vi "CRYExport to Excel with Close.vi"(4 "Format info":T1, 6 "ExcelPath":string, 8 "FilePath":string, 9 "Sheet Names":string[](array[string]), 10 "Data":string[][][](array[string]), 11 "New/Append":string) -> (0 "error out":errorcluster)   [LabVIEW 2013]
uses:
  <vilib>/addons/_office/_exclsub.llb/font.ctl
  <vilib>/Utility/NIReport.llb/NI_report.lvclass
  <vilib>/addons/_office/excel.llb/Excel Easy Table (str).vi
  <vilib>/Utility/NIReport.llb/Excel/NI_Excel.lvclass
  <vilib>/addons/_office/NI_ReportGenerationToolkit.lvlib
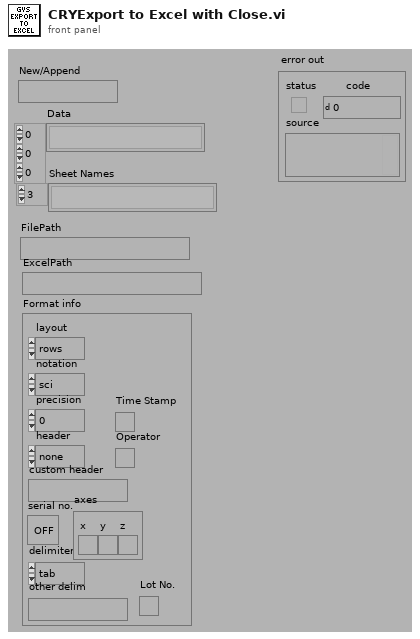
[diagram p1: front panel]
types:
  T1 = cluster{"layout":enum16{"rows", "columns"}, "notation":enum16{"sci", "float"}, "precision":i32, "header":enum16{"none", "standard", "custom"}, "custom header":string, "serial no.":bool, "delimiter":enum16{"tab", "comma", "space", "other"}, "other delim":string, "axes":cluster{"x":bool, "y":bool, "z":bool}, "Lot No.":bool, "Operator":bool, "Time Stamp":bool}
  T2 = typedef "NI_ReportGenerationToolkit.lvlib/font.ctl" = cluster{"font name":string, "font size":dbl, "bold":u16, "italic":u16, "underline":u16, "strike through":u16, "font color":u32}
  T3 = enum16{"OK", "Yes", "YesNo", "YesNoCancel", "ReplaceAppend"}
  T4 = enum16{"maximized", "minimized", "normal", "no change"}
  T5 = enum16{"Standard Report", "HTML", "Word", "Excel"}
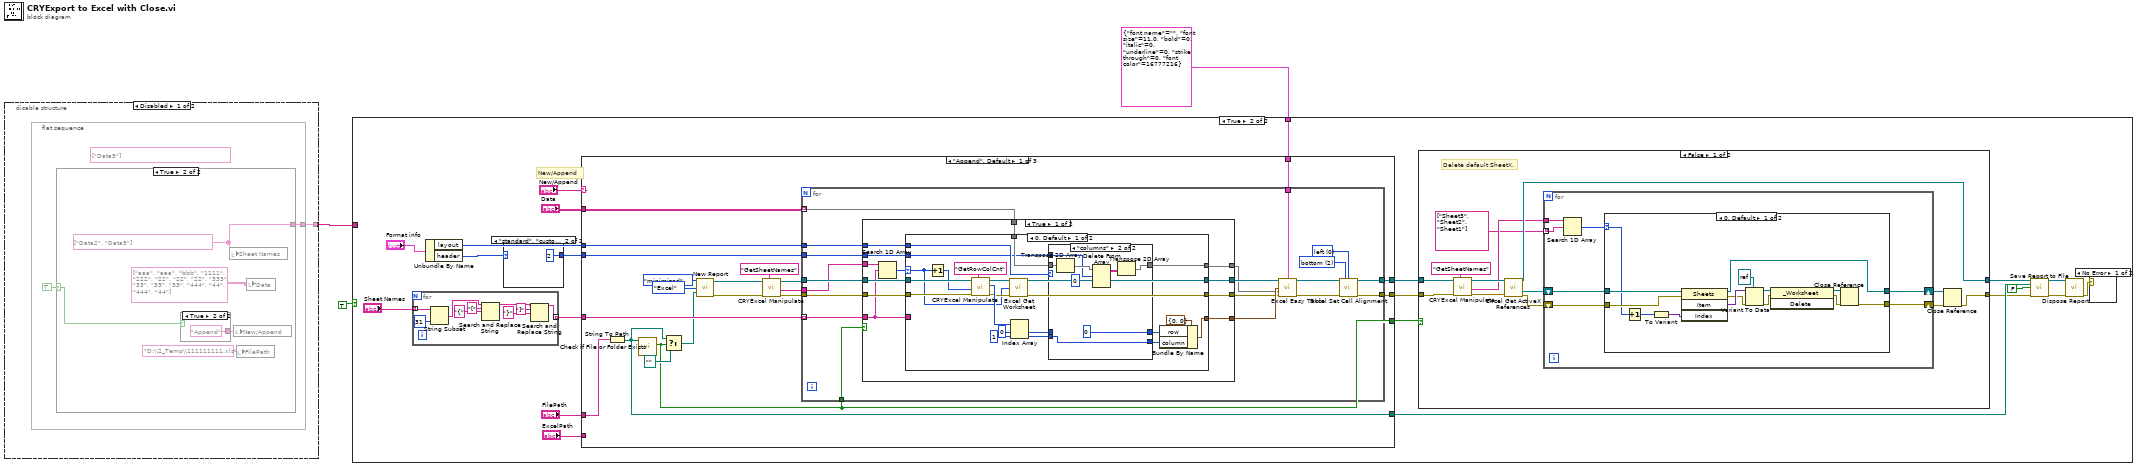
[diagram p0: block diagram]
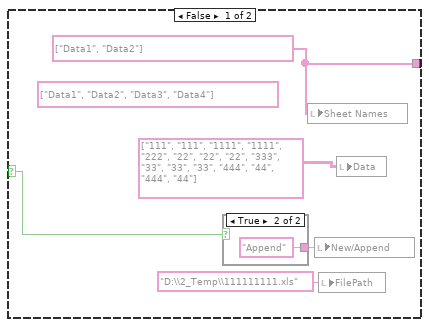
[diagram p2: hidden frame]
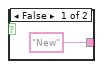
[diagram p3: hidden frame]
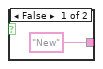
[diagram p4: hidden frame]
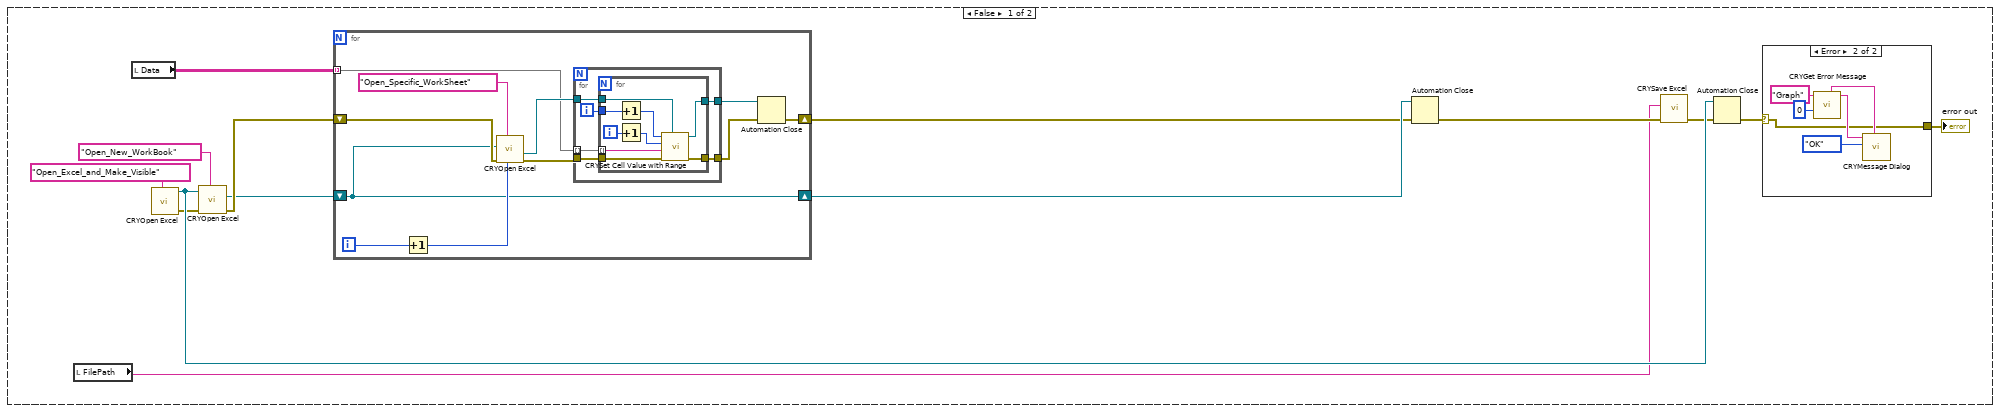
[diagram p6: hidden frame]
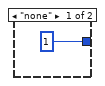
[diagram p8: hidden frame]
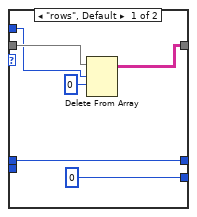
[diagram p12: hidden frame]
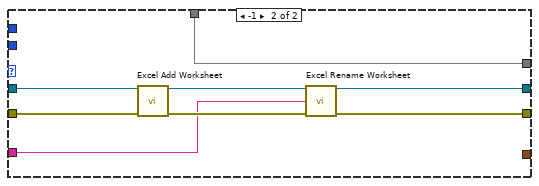
[diagram p13: hidden frame]
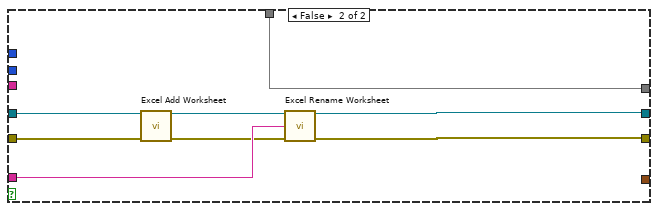
[diagram p14: hidden frame]
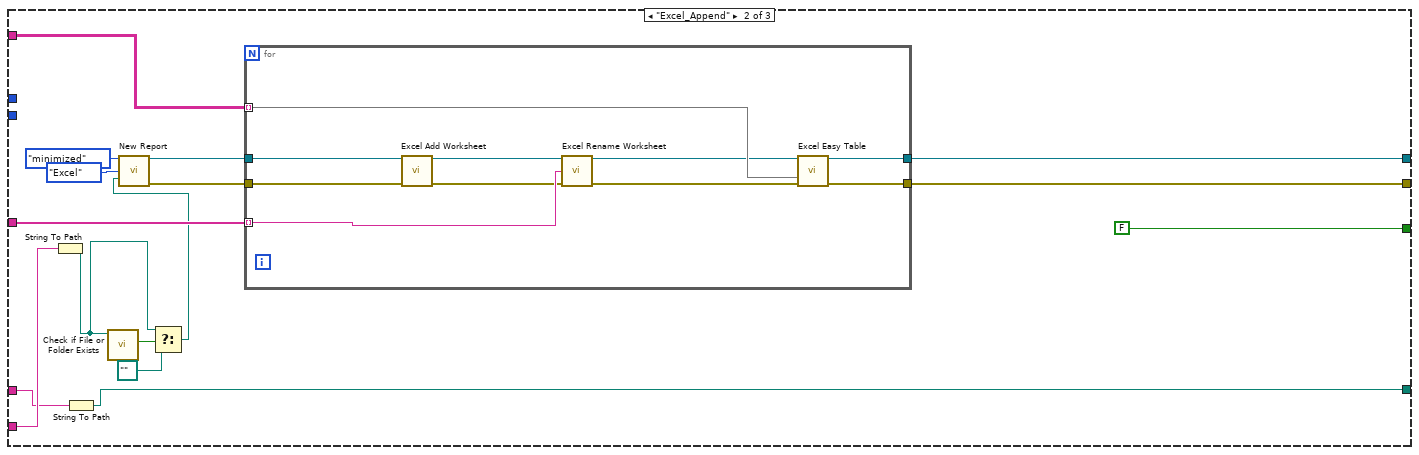
[diagram p15: hidden frame]
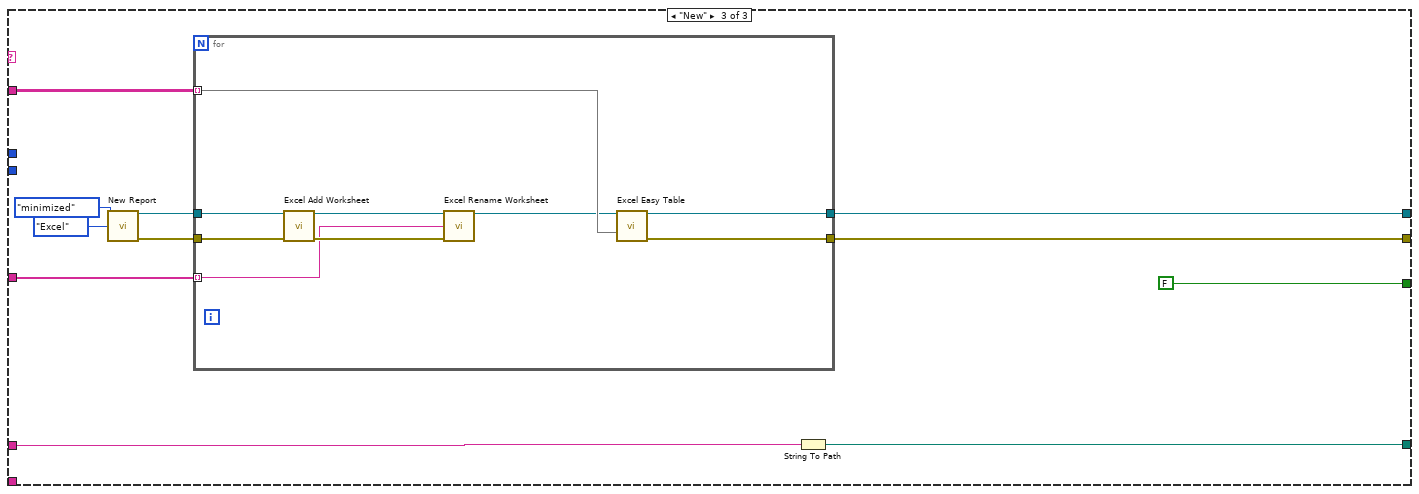
[diagram p16: hidden frame]
diagram:
  n1 = disable-structure shown="Disabled" {
    disable-tunnel: [w4 _] -> w2
    frame Disabled {
      n2 = flat-sequence {
        tunnel: [w6] -> w4
        frame #0 {
          (unwired) string[] ["Data5"] ("Data Names")
          n3 = case shown="True" TRUE {
            selector: TRUE -> [w8 w14]
            tunnel: [w7 w18] -> w6
            frame False {
              w7 = string[] ["Data1", "Data2"] ("Data Names")
              (unwired) string[] ["Data1", "Data2", "Data3", "Data4"] ("Data Names")
              n4 = case shown="True" w8 {
                tunnel: ["New" ("New/Append") "Append" ("New/Append")] -> w10
                frame False {
                }
                frame True {
                }
              }
              n5 = local write "Sheet Names"(w7) -> ()
              n6 = local write "New/Append"(w10) -> ()
              n7 = local write "FilePath"("D:\\2_Temp\\111111111.xls" ("FilePath")) -> ()
              n8 = local write "Data"(string[][][] [[["111", "111"], ["1111", "1111"]], [["222", "22"], ["22", "22"]], [["333", "33"], ["33", "33"]], [["444", "44"], ["444", "44"]]] ("appended array")) -> ()
            }
            frame True {
              w18 = string[] ["Data2", "Data5"] ("Data Names")
              n9 = case shown="True" w14 {
                tunnel: ["New" ("New/Append") "Append" ("New/Append")] -> w16
                frame False {
                }
                frame True {
                }
              }
              n10 = local write "Sheet Names"(w18) -> ()
              n11 = local write "New/Append"(w16) -> ()
              n12 = local write "FilePath"("D:\\2_Temp\\111111111.xls" ("FilePath")) -> ()
              n13 = local write "Data"(string[][][] [[["aaa", "aaa"], ["bbb", "1111"]], [["222", "22"], ["22", "22"]], [["333", "33"], ["33", "33"]], [["444", "44"], ["444", "44"]]] ("appended array")) -> ()
            }
          }
        }
      }
    }
    frame Enabled {
    }
  }
  n14 = case shown="True" TRUE {
    tunnel: w2 -> [_ _]
    tunnel: T2 {"font name"="", "font size"=11.0, "bold"=0, "italic"=0, "underline"=0, "strike through"=0, "font color"=16777216} ("font") -> [_ w72]
    frame False {
      n15 = local read "FilePath"() -> (w21:string)
      n16 = local read "Data"() -> (w22:string[][][])
      n17 = call "CRYOpen Excel.vi"("sActon"="Open_Excel_and_Make_Visible") -> ("error out"=w29:errorcluster, "Excel._Application out"=w32:refnum<k7>)  [unwired: 7 in, 2 out]
      n18 = call "CRYOpen Excel.vi"("sActon"="Open_New_WorkBook", "error in (no error)"=w29, "Excel._Application"=w32) -> ("error out"=w34:errorcluster, "Excel._Worksheets out"=w33:refnum<k7>)  [unwired: 5 in, 2 out]
      n19 = for {
        tunnel: w22 -> [w41] mode=indexing
        shift-right: [w35] -> w24
        shift-left: w34 -> [w45]
        shift-right: [w38] -> w25
        shift-left: w33 -> [w38]
        i -> [w40]
        n20 = Increment(x=w40) -> (x+1=w39:i32)
        n21 = call "CRYOpen Excel.vi"("Numeric"=w39, "sActon"="Open_Specific_WorkSheet", "error in (no error)"=w45, "Excel._Worksheets"=w38) -> ("error out"=w44:errorcluster, "Excel._Worksheet out"=w43:refnum<k7>)  [unwired: 4 in, 2 out]
        n22 = for {
          tunnel: w43 -> [w51]
          tunnel: w44 -> [w49]
          tunnel: [w48] -> w37
          tunnel: [w47] -> w36
          tunnel: w41 -> [w46] mode=indexing
          i -> [w50]
          n23 = for {
            tunnel: w51 -> [w59]
            tunnel: w49 -> [w58]
            tunnel: [w57] -> w47
            tunnel: w50 -> [w56]
            tunnel: [w55] -> w48
            tunnel: w46 -> [w52] mode=indexing
            i -> [w60]
            n24 = Increment(x=w56) -> (x+1=w54:i32)
            n25 = Increment(x=w60) -> (x+1=w53:i32)
            n26 = call "CRYSet Cell Value with Range.vi"("Excel._Worksheet"=w59, "error in (no error)"=w58, "Value"=w52, "Col"=w53, "Row"=w54) -> ("error out"=w57:errorcluster, "Excel._Worksheet"=w55:refnum<k7>)  [unwired: 2 out]
          }
        }
        n27 = Automation Close(3:w36, 5:w37) -> (0:w35:errorcluster)
      }
      n28 = Automation Close(3:w24, 5:w25) -> (0:w28:errorcluster)
      n29 = call "CRYSave Excel.vi"("error in (no error)"=w28, "FilePath"=w21) -> ("error out"=w27:errorcluster)  [unwired: 8 in]
      n30 = Automation Close(3:w27, 5:w32) -> (0:w26:errorcluster)
      n31 = case shown="Error" w26 {
        selector: w26 -> [w61 w62]
        tunnel: [w61 w62] -> w23
        frame No Error {
        }
        frame Error {
          n32 = call "CRYGet Error Message.vi"("Error No"=0, "Kind"="Graph") -> ("Message"=w64:string, "Window Title"=w63:string)  [unwired: 4 in, 4 out]
          n33 = call "CRYMessage Dialog.vi"("Window Title"=w63, "YesNoCancel"=T3."OK", "Message Content"=w64) -> ()  [unwired: 7 in, 2 out]
        }
      }
      "error out" <- w23
    }
    frame True {
      # "New/Append"
      n34 = for {
        tunnel: "Sheet Names" -> [w132] mode=indexing
        tunnel: [w129] -> w83 mode=indexing
        n35 = String Subset(string=w132, length (rest)=31 ("length (rest)")) -> (substring=w130:string)  [unwired: 1 in]
        n36 = Search and Replace String(input string=w130, search string="[", replace string="{" ("replace string (\"\")")) -> (result string=w133:string)  [unwired: 5 in, 3 out]
        n37 = Search and Replace String(input string=w133, search string="]", replace string="}" ("replace string (\"\")")) -> (result string=w129:string)  [unwired: 5 in, 3 out]
      }
      n38 = Unbundle By Name("Format info") -> ("layout"=w70:enum16{"rows", "columns"}, "header"=w69:enum16{"none", "standard", "custom"})
      n39 = case shown="\"standard\", \"custom\", Default" w69 {
        tunnel: [1 ("length") 2 ("length")] -> w68
        frame "none" {
        }
        frame "standard", "custom", Default {
        }
      }
      n40 = case shown="\"Append\", Default" "New/Append" {
        tunnel: "Data" -> [w156 w253 w274]
        tunnel: w83 -> [w155 w252 w273]
        tunnel: "FilePath" -> [w153 w247 w272]
        tunnel: "ExcelPath" -> [_ w248 _]
        tunnel: [w150 w243 w271] -> w79
        tunnel: [w149 w245 w270] -> w78
        tunnel: [w148 w244 w269] -> w77
        tunnel: [w151 FALSE ("file or folder exists?") FALSE] -> w74
        tunnel: w70 -> [w144 _ _]
        tunnel: w72 -> [w140 _ _]
        tunnel: w68 -> [w139 _ _]
        frame "Append", Default {
          n41 = String To Path(string=w153) -> (path=w150:path)
          n42 = call <vilib>:"Check if File or Folder Exists.vi"("path"=w150) -> ("file or folder exists?"=w151:bool)  [unwired: 8 in, 2 out]
          n43 = Select(t=w150, s=w151, f=path "") -> (s? t:f=w152:path)
          n44 = call <vilib>:"New Report.vi"("window state (normal)"=T4."minimized", "report type"=T5."Excel", "template (empty)"=w152) -> ("report out"=w143:refnum<class "NI_report.lvclass">, "error out"=w141:errorcluster)  [unwired: 3 in, 8 out]
          n45 = call "CRYExcel Manipulate.vi"("sAction"="GetSheetNames", "error in (no error)"=w141, "report in"=w143) -> ("error out"=w146:errorcluster, "sData out"=w145:string[], "report out"=w142:refnum<class "NI_report.lvclass">)  [unwired: 5 in, 1 out]
          n46 = for {
            tunnel: w142 -> [w176]
            tunnel: w146 -> [w175]
            tunnel: [w162] -> w149
            tunnel: [w160] -> w148
            tunnel: w156 -> [w167] mode=indexing
            tunnel: w155 -> [w174] mode=indexing
            tunnel: w151 -> [w173]
            tunnel: w145 -> [w172]
            tunnel: w144 -> [w168]
            tunnel: w140 -> [w165]
            tunnel: w139 -> [w164]
            w158 = 0 items=["left", "center", "right"] ("horizontal alignment (left)")
            w159 = 2 items=["top", "center", "bottom"] ("vertical alignment (top)")
            n47 = case shown="True" w173 {
              tunnel: w176 -> [w188 w240]
              tunnel: w175 -> [w187 w239]
              tunnel: [w186 w237] -> w170
              tunnel: [w185 w236] -> w169
              tunnel: w174 -> [w183 w238]
              tunnel: w172 -> [w184 _]
              tunnel: [w181 _] -> w171
              tunnel: w168 -> [w180 _]
              tunnel: [w179 w235] -> w166
              tunnel: w167 -> [w178 w235]
              tunnel: w164 -> [w177 _]
              frame True {
                n48 = Search 1D Array(1D array=w184, element=w183) -> (index of element=w182:i32)  [unwired: 1 in]
                n49 = case shown="0, Default" w182 {
                  selector: w182 -> [w190 _]
                  tunnel: w188 -> [w209 w232]
                  tunnel: w187 -> [w208 w231]
                  tunnel: [w193 w230] -> w186
                  tunnel: [w192 w229] -> w185
                  tunnel: w183 -> [_ w226]
                  tunnel: [w203 _] -> w181
                  tunnel: w180 -> [w202 _]
                  tunnel: [w196 w225] -> w179
                  tunnel: w178 -> [w197 w225]
                  tunnel: w177 -> [w189 _]
                  frame 0, Default {
                    n50 = Increment(x=w190) -> (x+1=w191:i32)
                    n51 = call "CRYExcel Manipulate.vi"("sAction"="GetRowColCnt", "error in (no error)"=w208, "nData"=w191, "report in"=w209) -> ("error out"=w194:errorcluster, "nData out"=w206:i32[], "report out"=w195:refnum<class "NI_report.lvclass">)  [unwired: 4 in, 1 out]
                    n52 = call <vilib>:"Excel Get Worksheet.vi"("report in"=w195, "worksheet index (0)"=w190, "error in (no error)"=w194) -> ("report out"=w193:refnum<class "NI_report.lvclass">, "error out"=w192:errorcluster)  [unwired: 1 in, 10 out]
                    n53 = Index Array(array=w206, index #1=0 ("index"), index #2=1 ("index")) -> (element #1=w201:i32, element #2=w200:i32)
                    n54 = case shown="\"columns\"" w202 {
                      tunnel: w201 -> [w215 _]
                      tunnel: w200 -> [_ w224]
                      tunnel: [0 ("column") w224] -> w199
                      tunnel: [w215 0 ("Count")] -> w198
                      tunnel: w197 -> [w213 w222]
                      tunnel: [w212 w218] -> w196
                      tunnel: w189 -> [w211 w217]
                      frame "rows", Default {
                        n55 = Delete From Array(array=w213, length=w211, index (row)=0 ("index")) -> (array with subset deleted=w212:string[][])  [unwired: 1 in, 1 out]
                      }
                      frame "columns" {
                        n56 = Transpose 2D Array(2D array=w222) -> (transposed array=w220:string[][])
                        n57 = Delete From Array(array=w220, length=w217, index (row)=0 ("index")) -> (array with subset deleted=w219:string[][])  [unwired: 1 in, 1 out]
                        n58 = Transpose 2D Array(2D array=w219) -> (transposed array=w218:string[][])
                      }
                    }
                    n59 = Bundle By Name(cluster=cluster{"row":i32, "column":i32} {"row"=0, "column"=0} ("start (0, 0)"), "row"=w198, "column"=w199) -> (w203:cluster{"row":i32, "column":i32})
                  }
                  frame -1 {
                    n60 = call <vilib>:"Excel Add Worksheet.vi"("report in"=w232, "error in (no error)"=w231) -> ("report out"=w228:refnum<class "NI_report.lvclass">, "error out"=w227:errorcluster)  [unwired: 12 out]
                    n61 = call <vilib>:"Excel Rename Worksheet.vi"("report in"=w228, "worksheet name (\"\")"=w226, "error in (no error)"=w227) -> ("report out"=w230:refnum<class "NI_report.lvclass">, "error out"=w229:errorcluster)  [unwired: 11 out]
                  }
                }
              }
              frame False {
                n62 = call <vilib>:"Excel Add Worksheet.vi"("report in"=w240, "error in (no error)"=w239) -> ("report out"=w234:refnum<class "NI_report.lvclass">, "error out"=w233:errorcluster)  [unwired: 12 out]
                n63 = call <vilib>:"Excel Rename Worksheet.vi"("report in"=w234, "worksheet name (\"\")"=w238, "error in (no error)"=w233) -> ("report out"=w237:refnum<class "NI_report.lvclass">, "error out"=w236:errorcluster)  [unwired: 11 out]
              }
            }
            n64 = call-poly <vilib>:"Excel Easy Table.vi"("report in"=w170, "font"=w165, "start (0, 0)"=w171, "text data"=w166, "error in (no error)"=w169) -> ("report out"=w163:refnum<class "NI_report.lvclass">, "error out"=w161:errorcluster)  [unwired: 4 in, 5 out]
            n65 = call <vilib>:"Excel Set Cell Alignment.vi"("report in"=w163, "vertical alignment (top)"=w159, "horizontal alignment (left)"=w158, "error in (no error)"=w161) -> ("report out"=w162:refnum<class "NI_report.lvclass">, "error out"=w160:errorcluster)  [unwired: 10 in]
          }
        }
        frame "Excel_Append" {
          n66 = String To Path(string=w248) -> (path=w246:path)
          n67 = String To Path(string=w247) -> (path=w243:path)
          n68 = call <vilib>:"Check if File or Folder Exists.vi"("path"=w246) -> ("file or folder exists?"=w250:bool)  [unwired: 8 in, 2 out]
          n69 = Select(t=w246, s=w250, f=path "") -> (s? t:f=w249:path)
          n70 = call <vilib>:"New Report.vi"("window state (normal)"=T4."minimized", "report type"=T5."Excel", "template (empty)"=w249) -> ("report out"=w254:refnum<class "NI_report.lvclass">, "error out"=w255:errorcluster)  [unwired: 3 in, 8 out]
          n71 = for {
            tunnel: w254 -> [w263]
            tunnel: w255 -> [w262]
            tunnel: [w266] -> w245
            tunnel: [w265] -> w244
            tunnel: w253 -> [w264] mode=indexing
            tunnel: w252 -> [w260] mode=indexing
            n72 = call <vilib>:"Excel Add Worksheet.vi"("report in"=w263, "error in (no error)"=w262) -> ("report out"=w258:refnum<class "NI_report.lvclass">, "error out"=w257:errorcluster)  [unwired: 12 out]
            n73 = call <vilib>:"Excel Rename Worksheet.vi"("report in"=w258, "worksheet name (\"\")"=w260, "error in (no error)"=w257) -> ("report out"=w261:refnum<class "NI_report.lvclass">, "error out"=w259:errorcluster)  [unwired: 11 out]
            n74 = call-poly <vilib>:"Excel Easy Table.vi"("report in"=w261, "text data"=w264, "error in (no error)"=w259) -> ("report out"=w266:refnum<class "NI_report.lvclass">, "error out"=w265:errorcluster)  [unwired: 5 in, 6 out]
          }
        }
        frame "New" {
          n75 = call <vilib>:"New Report.vi"("window state (normal)"=T4."minimized", "report type"=T5."Excel") -> ("report out"=w275:refnum<class "NI_report.lvclass">, "error out"=w276:errorcluster)  [unwired: 4 in, 8 out]
          n76 = for {
            tunnel: w275 -> [w281]
            tunnel: w276 -> [w279]
            tunnel: [w286] -> w270
            tunnel: [w285] -> w269
            tunnel: w274 -> [w284] mode=indexing
            tunnel: w273 -> [w278] mode=indexing
            n77 = call <vilib>:"Excel Add Worksheet.vi"("report in"=w281, "error in (no error)"=w279) -> ("report out"=w283:refnum<class "NI_report.lvclass">, "error out"=w282:errorcluster)  [unwired: 12 out]
            n78 = call <vilib>:"Excel Rename Worksheet.vi"("report in"=w283, "worksheet name (\"\")"=w278, "error in (no error)"=w282) -> ("report out"=w280:refnum<class "NI_report.lvclass">)  [unwired: 12 out]
            n79 = call-poly <vilib>:"Excel Easy Table.vi"("report in"=w280, "text data"=w284) -> ("report out"=w286:refnum<class "NI_report.lvclass">, "error out"=w285:errorcluster)  [unwired: 6 in, 6 out]
          }
          n80 = String To Path(string=w272) -> (path=w271:path)
        }
      }
      n81 = case shown="False" w74 {
        tunnel: w78 -> [w103 w128]
        tunnel: w77 -> [w102 w127]
        tunnel: [w101 w128] -> w76
        tunnel: [w100 w127] -> w75
        frame False {
          # "Delete default SheetX."
          n82 = call "CRYExcel Manipulate.vi"("sAction"="GetSheetNames", "error in (no error)"=w102, "report in"=w103) -> ("error out"=w93:errorcluster, "sData out"=w92:string[], "report out"=w94:refnum<class "NI_report.lvclass">)  [unwired: 5 in, 1 out]
          n83 = call <vilib>:"Excel Get ActiveX References.vi"("report in"=w94, "error in (no error)"=w93) -> ("report out"=w101:refnum<class "NI_report.lvclass">, "Excel.Sheets"=w99:refnum<k7>, "error out"=w98:errorcluster)  [unwired: 7 in, 4 out]
          n84 = for {
            shift-right: [w108] -> w96
            shift-left: w98 -> [w107]
            shift-right: [w109] -> w97
            shift-left: w99 -> [w110]
            tunnel: w92 -> [w105]
            tunnel: string[] ["Sheet3", "Sheet2", "Sheet1"] ("sData out") -> [w104] mode=indexing
            n85 = Search 1D Array(1D array=w105, element=w104) -> (index of element=w106:i32)  [unwired: 1 in]
            n86 = case shown="0, Default" w106 {
              selector: w106 -> [w112 _]
              tunnel: w110 -> [w120 w126]
              tunnel: [w118 w126] -> w109
              tunnel: [w117 w125] -> w108
              tunnel: w107 -> [w116 w125]
              frame 0, Default {
                n87 = Increment(x=w112) -> (x+1=w111:i32)
                n88 = To Variant(anything=w111) -> (Variant=w119:variant)
                n89 = invoke class="Sheets" method="Item"(reference=w120, error in=w116, "Index"=w119) -> (reference out=w118:refnum<k7>, error out=w115:errorcluster, "Item"=w124:variant)  [unwired: 1 in, 1 out]
                n90 = Variant To Data(error in=w115, type=refnum<k7> refnum ("Worksheets"), Variant=w124) -> (data=w122:refnum<k7>, error out=w114:errorcluster)
                n91 = invoke class="_Worksheet" method="Delete"(reference=w122, error in=w114) -> (reference out=w121:refnum<k7>, error out=w113:errorcluster)  [unwired: 1 in, 1 out]
                n92 = Close Reference(reference=w121, error in (no error)=w113) -> (error out=w117:errorcluster)
              }
              frame -1 {
              }
            }
          }
          n93 = Close Reference(reference=w97, error in (no error)=w96) -> (error out=w100:errorcluster)
        }
        frame True {
        }
      }
      n94 = call-dynamic "Save Report to File.vi"("report in"=w76, "report file path"=w79, "prompt to replace? (F)"=FALSE, "error in (no error)"=w75) -> ("report out"=w81:refnum<class "NI_report.lvclass">, "error out"=w82:errorcluster)  [unwired: 10 in]
      n95 = call-dynamic "Dispose Report.vi"("report in"=w81, "error in (no error)"=w82) -> ("error out"=w73:errorcluster)  [unwired: 13 in]
      n96 = case shown="No Error" w73 {
        frame No Error {
        }
        frame Error {
        }
      }
    }
  }
